vi "StopRequest.vi"(8 "ErrorArray In":errorcluster[](array[cluster]), 11 "BusIndex":i8=-1) -> (0 "ErrorArray Out":errorcluster[](array[cluster]))   [LabVIEW 2014, in "Framework.lvlib"]
uses:
  Framework.lvlib
  <vilib>/event_ctls.llb/usereventprio.ctl
  Protected/clUserEventType.ctl
  <userlib>/NIST/NISTErrorLib/NISTErrorLib.lvlib
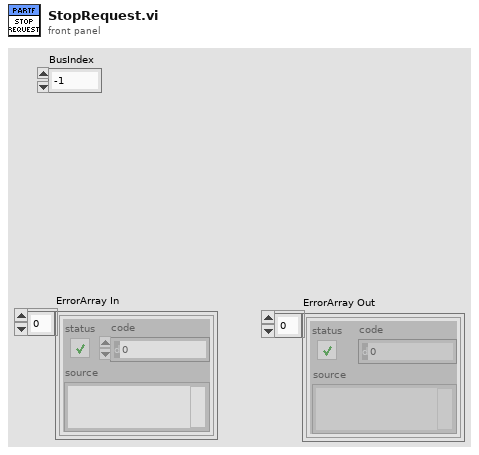
[diagram p1: front panel]
types:
  T1 = typedef "Framework.lvlib/clUserEventType.ctl" = cluster{"BusIndex":i8, "Data":variant}
  T2 = typedef "usereventprio.ctl" = enum32{"high priority", "normal priority"}
  T3 = typedef "Framework.lvlib/clRequestEvents.ctl" = cluster{"StopRequest":refnum<user-event>}
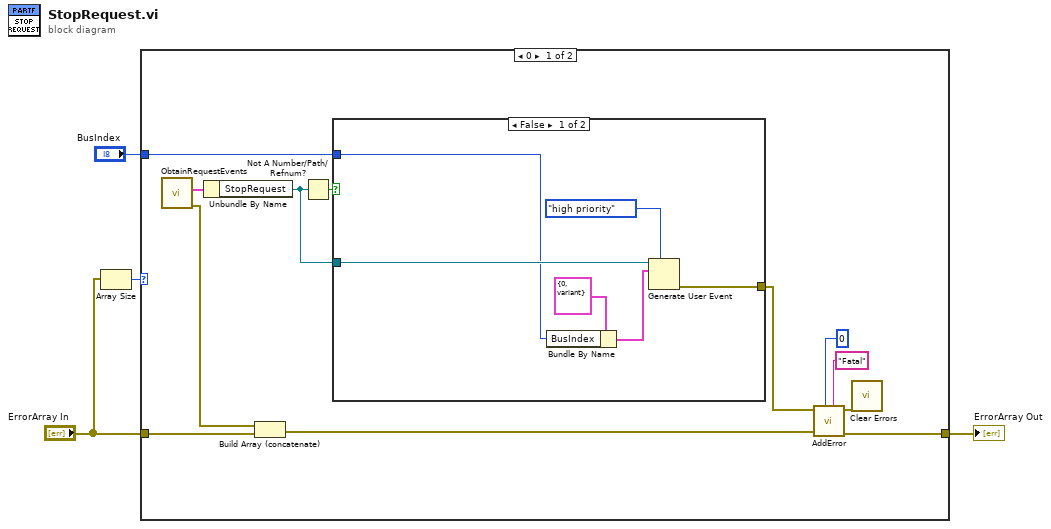
[diagram p0: block diagram]
diagram:
  n1 = Array Size(array="ErrorArray In") -> (size(s)=w3:i32)
  n2 = case shown="0" w3 {
    tunnel: "ErrorArray In" -> [w16 w23]
    tunnel: [w15 w23] -> w4
    tunnel: "BusIndex" -> [w7 _]
    frame 0 {
      n3 = call "ObtainRequestEvents.vi"() -> ("ErrorArray Out"=w5:errorcluster[], "clRequestEvents"=w11:T3)  [unwired: 10 in]
      n4 = Unbundle By Name(w11) -> ("StopRequest"=w9:refnum<user-event>)
      n5 = Build Array (concatenate)(w5, w16) -> (w6:errorcluster[])
      n6 = Not A Number/Path/Refnum?(number/path/refnum=w9) -> (NaN/Path/Refnum?=w10:bool)
      n7 = case shown="False" w10 {
        tunnel: w9 -> [w21 _]
        tunnel: [w20 _] -> w8
        tunnel: w7 -> [w17 _]
        frame False {
          n8 = Bundle By Name(cluster=T1 {"BusIndex"=0, "Data"=variant} ("clEventType"), "BusIndex"=w17) -> (w18:T1)
          n9 = Generate User Event(priority (normal)=usereventprio."high priority", user event=w21, event data cluster=w18) -> (error out=w20:errorcluster)  [unwired: 1 in, 1 out]
        }
        frame True {
        }
      }
      n10 = call <userlib>:"AddError.vi"("Severity"="Fatal" ("String"), "Priority"=u8 0, "ErrorArray"=w6, "error in (no error)"=w8) -> ("ErrorArray"=w15:errorcluster[], "error out"=w14:errorcluster)  [unwired: 6 in]
      n11 = call <vilib>:"Clear Errors.vi"("error in (no error)"=w14) -> ()  [unwired: 5 in, 2 out]
    }
    frame 1, Default {
    }
  }
  "ErrorArray Out" <- w4
